vi "Init.vi"(7 "Enclave":refnum<class "Enclave.lvclass">, 11 "Queue":refnum<queue>) -> (3 "Lossless out":refnum<class "Lossless.lvclass">)   [LabVIEW 2022 SP3, in "Enclave.lvlib" / "Lossless.lvclass"]
uses:
  Lossless.lvclass
  Enclave/Enclave.lvclass
  Element.ctl
  Lossless.lvclass/Lossless.ctl
  Enclave.lvlib
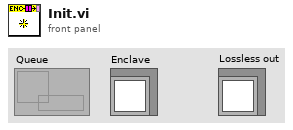
[diagram p1: front panel]
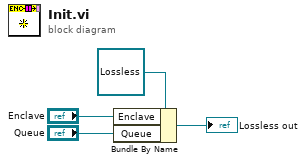
[diagram p0: block diagram]
diagram:
  n1 = Bundle By Name(cluster=refnum<class "Lossless.lvclass"> refnum ("Lossless in"), "Enclave"="Enclave", "Queue"="Queue") -> (→"Lossless out":refnum<class "Lossless.lvclass">)
